vi "newFrame.vi"(6 "Frame Instruction 3":T1={"Code Rates"=4.0, "Length"=12.0, "Destination address"=8.0, "User"=2.0, "Source address "=8.0, " Frame number"=8.0, " Check sum"=16.0}, 8 "Modulation type":dbl, 10 "Frame number":dbl) -> (1 "symbols":cdb[](array[numeric]) format="%.3f")   [LabVIEW 2014]
uses:
  <vilib>/addons/Modulation/Digital/General/MT Generate Bits (Galois, PN Order).vi
  <vilib>/addons/Modulation/Digital/Support/Common/Validators/mod_Generate Bits Validate.vi
  <vilib>/addons/Modulation/Analog/support/mod_Set Error Source.vi
  <vilib>/addons/Modulation/Digital/General/subVIs/mod_Generate Bits PN Sequence.vi
  <vilib>/addons/Modulation/Digital/General/MT Map Bits to PSK Symbols.vi
  <vilib>/addons/Modulation/niDMT.lvlib
panel:
  out "size(s)":i32
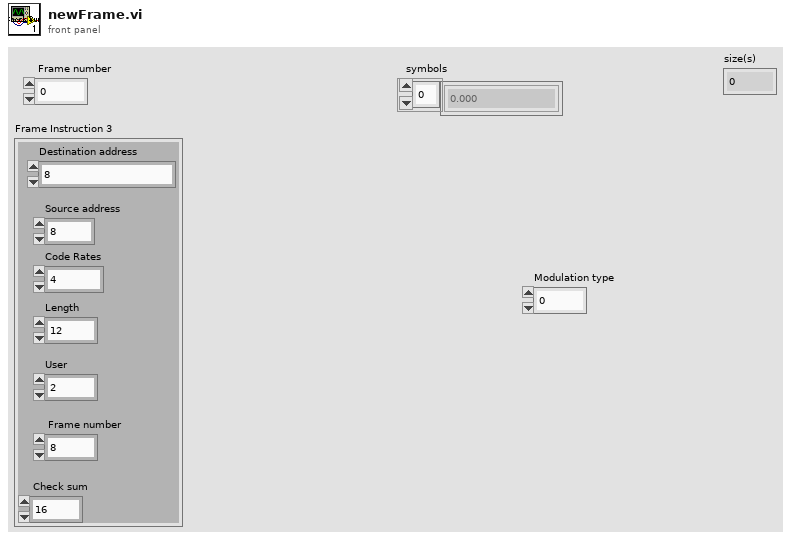
[diagram p1: front panel]
types:
  T1 = cluster{"Code Rates":dbl, "Length":dbl, "Destination address":dbl, "User":dbl, "Source address ":dbl, " Frame number":dbl, " Check sum":dbl}
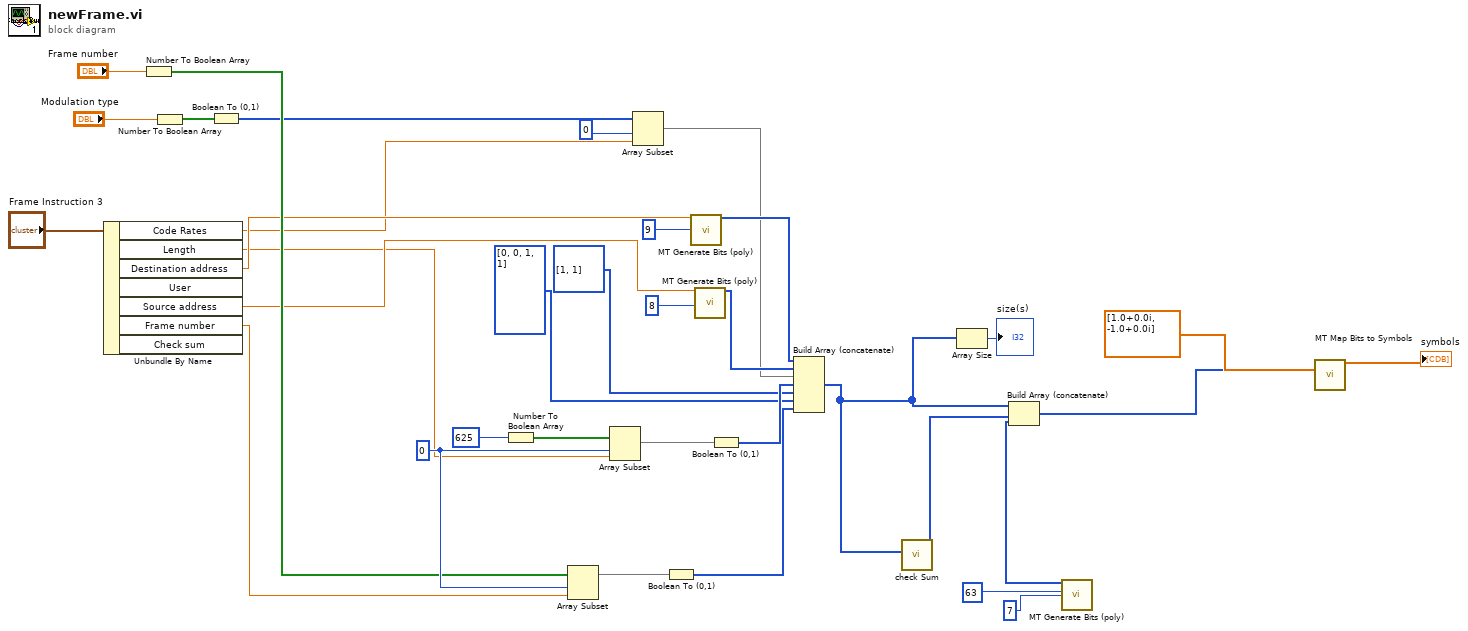
[diagram p0: block diagram]
diagram:
  w22 = 0
  n1 = Unbundle By Name("Frame Instruction 3") -> ("Code Rates"=w8:dbl, "Length"=w12:dbl, "Destination address"=w14:dbl, "Source address"=w13:dbl, "Frame number"=w11:dbl)  [unwired: 2 out]
  n2 = Number To Boolean Array(number="Frame number") -> (Boolean array=w15:bool[])
  n3 = Number To Boolean Array(number="Modulation type") -> (Boolean array=w33:bool[])
  n4 = Boolean To (0,1)(Boolean=w33) -> (0, 1=w10:i16[])
  n5 = Number To Boolean Array(number=625) -> (Boolean array=w29:bool[])
  n6 = Array Subset(array=w15, index=w22, length=w11) -> (w21:bool[])
  n7 = Array Subset(array=w29, index=w22, length=w12) -> (w28:bool[])
  n8 = Array Subset(array=w10, index=0, length=w8) -> (w3:i16[])
  n9 = Boolean To (0,1)(Boolean=w21) -> (0, 1=w16:i16[])
  n10 = call-poly <vilib>:"MT Generate Bits (poly).vi"("total bits (128)"=w14, "PN sequence order (9)"=9) -> ("output bit stream"=w26:i8[])  [unwired: 11 in, 2 out]
  n11 = call-poly <vilib>:"MT Generate Bits (poly).vi"("total bits (128)"=w13, "PN sequence order (9)"=8) -> ("output bit stream"=w23:i8[])  [unwired: 11 in, 2 out]
  n12 = Boolean To (0,1)(Boolean=w28) -> (0, 1=w27:i16[])
  n13 = Build Array (concatenate)(w26, w23, w3, w27, i32[] [1, 1], i32[] [0, 0, 1, 1], w16) -> (w1:i32[])
  n14 = call "check Sum.vi"("Array"=w1) -> ("subarray"=w18:i32[])  [unwired: 10 in]
  n15 = Array Size(array=w1) -> (size(s)=→"size(s)":i32)
  n16 = call-poly <vilib>:"MT Generate Bits (poly).vi"("total bits (128)"=63, "PN sequence order (9)"=7) -> ("output bit stream"=w5:i8[])  [unwired: 11 in, 2 out]
  n17 = Build Array (concatenate)(w1, w18, w5) -> (w4:i32[])
  n18 = call-poly <vilib>:"MT Map Bits to Symbols.vi"("input bit stream"=w4, "symbol map"=cdb[] [1.0+0.0i, -1.0+0.0i]) -> ("symbols"=→"symbols":cdb[])  [unwired: 12 in, 1 out]
